vi "test_PhotonCamera_EmptyResult.vi"(8 "error in (no error)":errorcluster) -> (0 "error out":errorcluster, 3 "Test Passed":bool)   [LabVIEW 2019]
uses:
  <vilib>/Rock Robotics/WPI/ThirdParty/PhotonVisionLib/PhotonVisionLib.lvlib
  <vilib>/Rock Robotics/WPI/ThirdParty/PhotonVisionLib/TypeDef/TargetCornerType.ctl
  <vilib>/Rock Robotics/WPI/ThirdParty/PhotonVisionLib/TypeDef/PhotonTrackedTargetType.ctl
  <vilib>/Rock Robotics/WPI/ThirdParty/PhotonVisionLib/TypeDef/PhotonPipelineResultType.ctl
  <vilib>/Rock Robotics/WPI/ThirdParty/JAS_Junk/TrajLib/TypeDef/TRANSLATION3D.ctl
  <vilib>/Rock Robotics/WPI/ThirdParty/JAS_Junk/TrajLib/Trajectory_Library.lvlib
  <vilib>/Rock Robotics/WPI/ThirdParty/JAS_Junk/TrajLib/TypeDef/QUATERNION.ctl
  <vilib>/Rock Robotics/WPI/ThirdParty/JAS_Junk/TrajLib/TypeDef/ROTATION3D.ctl
  <vilib>/Rock Robotics/WPI/ThirdParty/JAS_Junk/TrajLib/TypeDef/TRANSFORM3D.ctl
  <vilib>/Rock Robotics/WPI/ThirdParty/PhotonVisionLib/TypeDef/PhotonPNPResultType.ctl
  <vilib>/Rock Robotics/WPI/ThirdParty/PhotonVisionLib/TypeDef/PhotonMultiTargetPNPResultType.ctl
  <vilib>/Rock Robotics/WPI/ThirdParty/PhotonVisionLib/TypeDef/PhotonPipelineMetadataType.ctl
panel:
  out "PhotonPipelineResult":T1={"Targets"=[], "PhotonMultiTargetPNPResult"={"PhotonPNPResult"={"IsPresent"=FALSE, "bestReprojErr"=0.0, "altReprojErr"=0.0, "ambiguity"=0.0, "Best"={"TRANSLATION3D"={"X"=0.0, "Y"=0.0, "Z"=0.0}, "ROTATION3D"={"Q_quaternion"={"R"=1.0, "V"=[0.0, 0.0, 0.0]}}, "XF"=FALSE}, "Alt"={"TRANSLATION3D"={"X"=0.0, "Y"=0.0, "Z"=0.0}, "ROTATION3D"={"Q_quaternion"={"R"=1.0, "V"=[0.0, 0.0, 0.0]}}, "XF"=FALSE}}, "FiducialIDsUsed"=[]}, "PhotonPipelineMetadata"={"CaptureTimestampMicros"=0, "PublishTimestampMicros"=0, "SequenceID"=0, "TimeSinceLastPong"=0}} {"PhotonMultiTargetPNPResult"."PhotonPNPResult"."Alt"."TRANSLATION3D"."Z" format="%14.3f"; "PhotonMultiTargetPNPResult"."PhotonPNPResult"."Alt"."TRANSLATION3D"."Y" format="%14.3f"; "PhotonMultiTargetPNPResult"."PhotonPNPResult"."Alt"."TRANSLATION3D"."X" format="%14.3f"; "PhotonMultiTargetPNPResult"."PhotonPNPResult"."Best"."TRANSLATION3D"."Z" format="%14.3f"; "PhotonMultiTargetPNPResult"."PhotonPNPResult"."Best"."TRANSLATION3D"."Y" format="%14.3f"; "PhotonMultiTargetPNPResult"."PhotonPNPResult"."Best"."TRANSLATION3D"."X" format="%14.3f"; "Targets"."AltCameraToTarget"."TRANSLATION3D"."Z" format="%14.3f"; "Targets"."AltCameraToTarget"."TRANSLATION3D"."Y" format="%14.3f"; "Targets"."AltCameraToTarget"."TRANSLATION3D"."X" format="%14.3f"; "Targets"."BestCameraToTarget"."TRANSLATION3D"."Z" format="%14.3f"; "Targets"."BestCameraToTarget"."TRANSLATION3D"."Y" format="%14.3f"; "Targets"."BestCameraToTarget"."TRANSLATION3D"."X" format="%14.3f"}
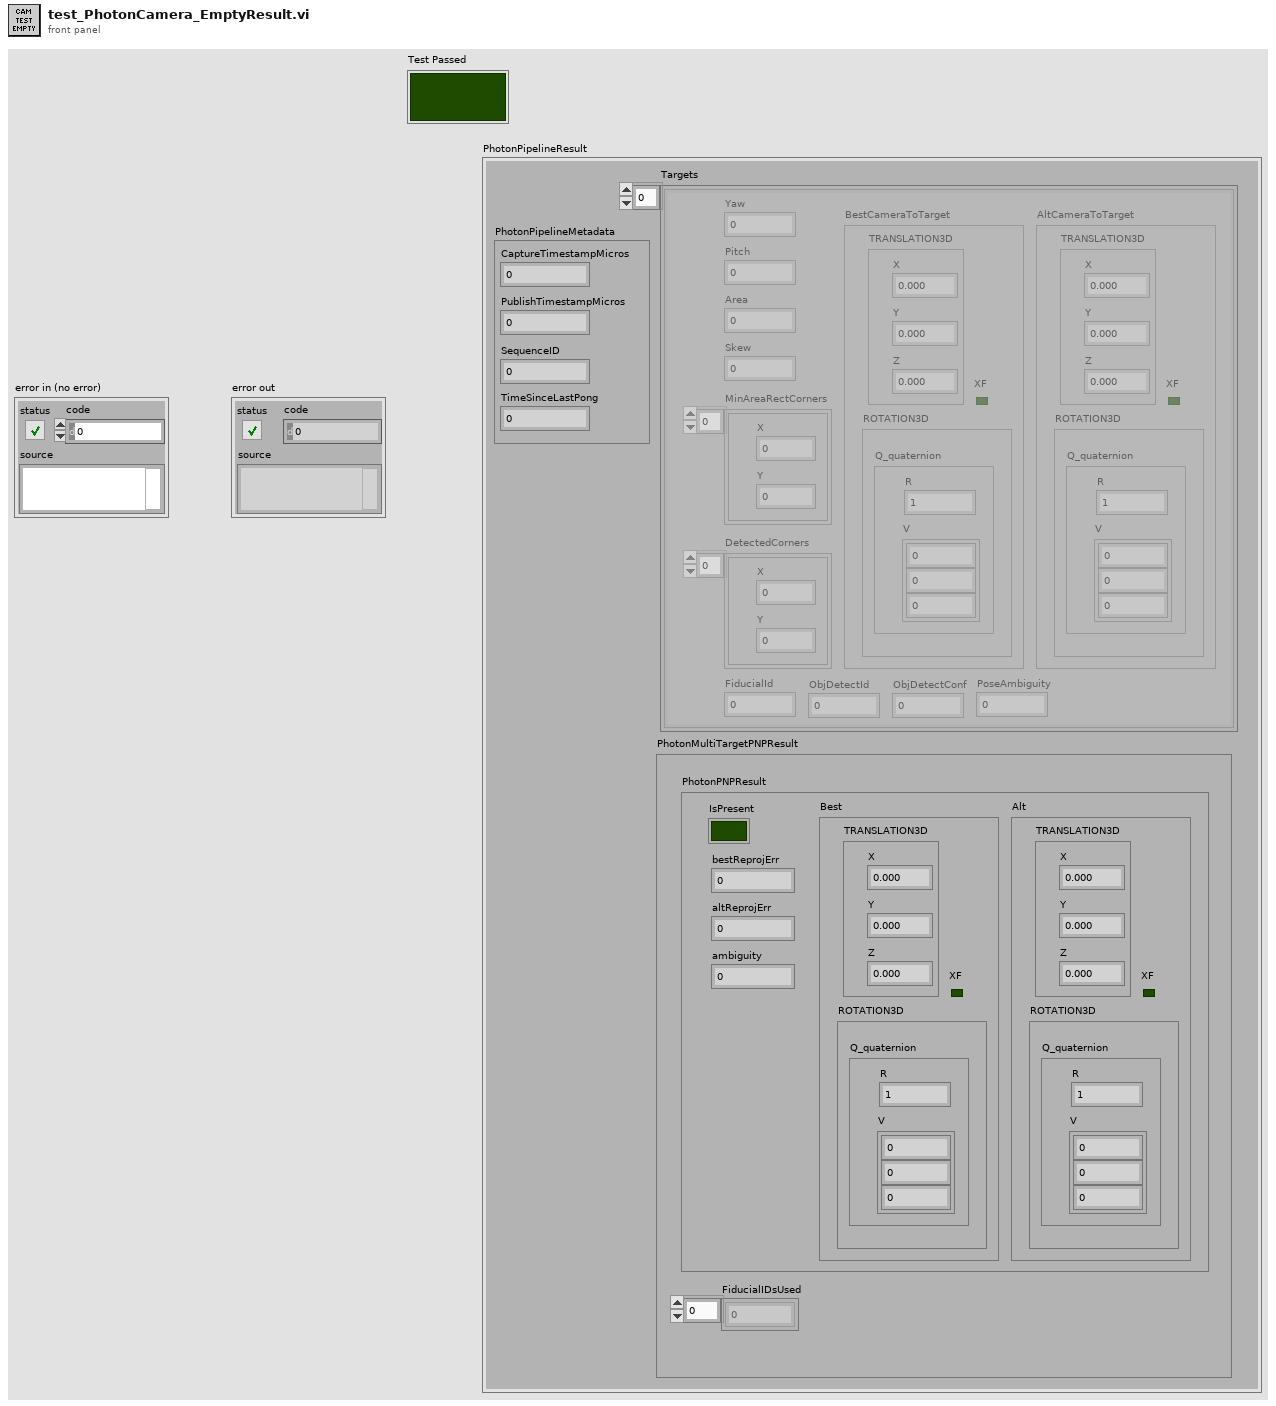
[diagram p1: front panel]
types:
  T1 = typedef "PhotonVisionLib.lvlib/PhotonPipelineResultType.ctl" = cluster{"Targets":T2[], "PhotonMultiTargetPNPResult":T8, "PhotonPipelineMetadata":T10}
  T2 = typedef "PhotonVisionLib.lvlib/PhotonTrackedTargetType.ctl" = cluster{"Yaw":dbl, "Pitch":dbl, "Area":dbl, "Skew":dbl, "MinAreaRectCorners":T3[], "BestCameraToTarget":T4, "FiducialId":i32, "AltCameraToTarget":T4, "PoseAmbiguity":dbl, "DetectedCorners":T3[], "ObjDetectId":i32, "ObjDetectConf":sgl}
  T3 = typedef "PhotonVisionLib.lvlib/TargetCornerType.ctl" = cluster{"X":dbl, "Y":dbl}
  T4 = typedef "Trajectory_Library.lvlib/TRANSFORM3D.ctl" = cluster{"TRANSLATION3D":T5, "ROTATION3D":T6, "XF":bool}
  T5 = typedef "Trajectory_Library.lvlib/TRANSLATION3D.ctl" = cluster{"X":dbl, "Y":dbl, "Z":dbl}
  T6 = typedef "Trajectory_Library.lvlib/ROTATION3D.ctl" = cluster{"Q_quaternion":T7}
  T7 = typedef "Trajectory_Library.lvlib/QUATERNION.ctl" = cluster{"R":dbl, "V":dbl[]}
  T8 = typedef "PhotonVisionLib.lvlib/PhotonMultiTargetPNPResultType.ctl" = cluster{"PhotonPNPResult":T9, "FiducialIDsUsed":i16[]}
  T9 = typedef "PhotonVisionLib.lvlib/PhotonPNPResultType.ctl" = cluster{"IsPresent":bool, "bestReprojErr":dbl, "altReprojErr":dbl, "ambiguity":dbl, "Best":T4, "Alt":T4}
  T10 = typedef "PhotonVisionLib.lvlib/PhotonPipelineMetadataType.ctl" = cluster{"CaptureTimestampMicros":i64, "PublishTimestampMicros":i64, "SequenceID":i64, "TimeSinceLastPong":i64}
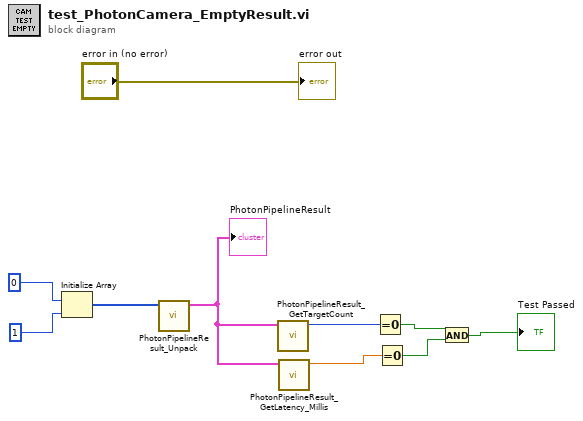
[diagram p0: block diagram]
diagram:
  n1 = Initialize Array(u8 0 ("Byte"), 1 ("dimension size")) -> (w7:u8[])
  n2 = call <vilib>:"PhotonPipelineResult_Unpack.vi"("RawData"=w7) -> ("PhotonPipelineResult"=w3:T1)  [unwired: 9 in, 1 out]
  "PhotonPipelineResult" <- w3
  n3 = call <vilib>:"PhotonPipelineResult_GetTargetCount.vi"("PhotonPipelineResult"=w3) -> ("TargetCount"=w2:i32)  [unwired: 10 in]
  n4 = call <vilib>:"PhotonPipelineResult_GetLatency_Millis.vi"("PhotonPipelineResult"=w3) -> ("Latency_MilliSec"=w1:dbl)  [unwired: 9 in, 1 out]
  n5 = Equal To 0?(x=w2) -> (x = 0?=w6:bool)
  n6 = Equal To 0?(x=w1) -> (x = 0?=w5:bool)
  n7 = And(x=w6, y=w5) -> (x .and. y?=→"Test Passed":bool)
  "error out" <- "error in (no error)"
